vi "Read Decimal and Octal Label Tags.vi"(8 "error in":errorcluster, 11 "node in":refnum<k20>) -> (0 "error out":errorcluster, 1 "label (Dec)":u32, 2 "label (Display)":u32, 3 "node out":refnum<k20>)   [LabVIEW 2020, in "ARINC 429 Import.lvlib"]
uses:
  ARINC 429 Import.lvlib
  <vilib>/xml/NI_XML.lvlib
  <resource>/objmgr/DOMUserDefRef.rc
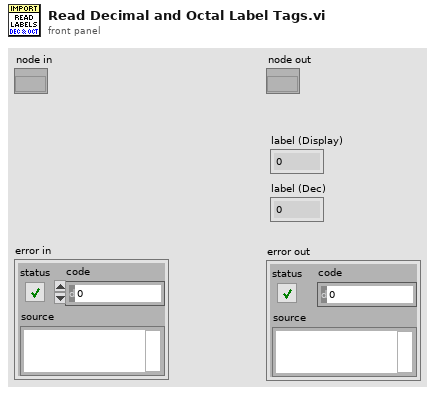
[diagram p1: front panel]
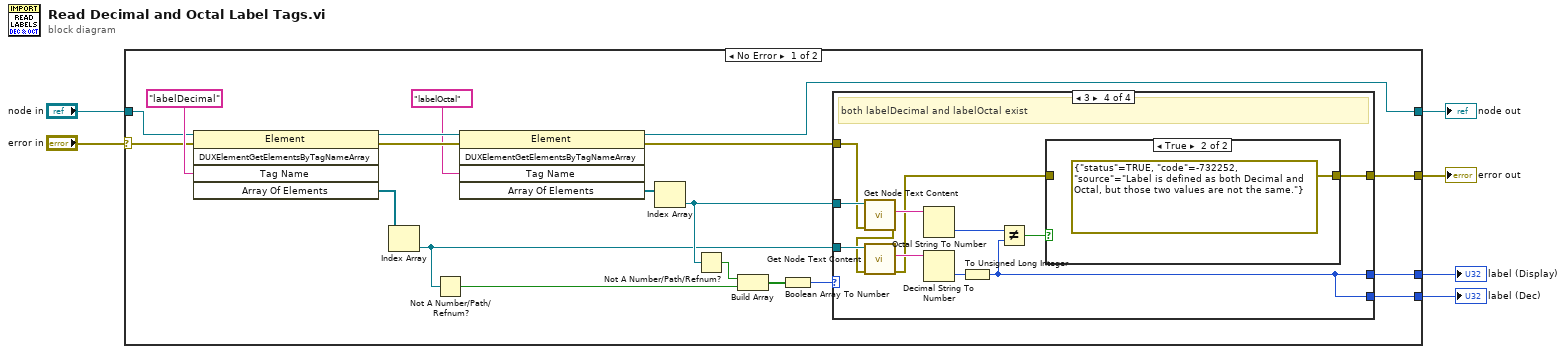
[diagram p0: block diagram]
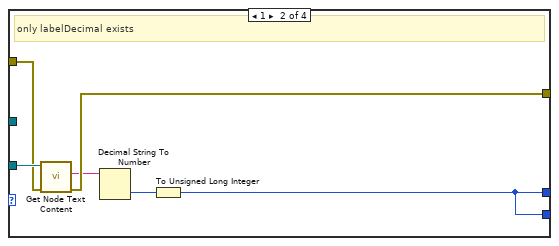
[diagram p3: hidden frame]
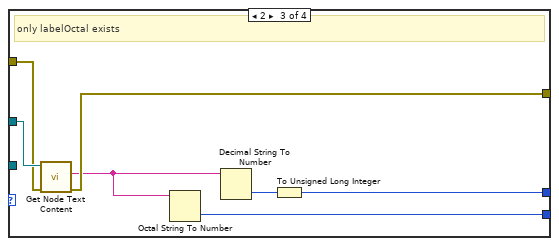
[diagram p4: hidden frame]
diagram:
  n1 = case shown="No Error" "error in" {
    selector: "error in" -> [w10 w55]
    tunnel: [w8 w55] -> w6
    tunnel: "node in" -> [w11 w54]
    tunnel: [w12 w54] -> w4
    tunnel: [w9 _] -> w2
    tunnel: [w7 _] -> w1
    frame No Error {
      n2 = invoke class="Element" method="DUXElementGetElementsByTagNameArray"(reference=w11, error in=w10, "Tag Name"="labelDecimal") -> (reference out=w17:refnum<k20>, error out=w18:errorcluster, "Array Of Elements"=w14:refnum<k20>[])  [unwired: 2 in, 2 out]
      n3 = Index Array(array=w14) -> (element=w23:refnum<k20>)  [unwired: 1 in]
      n4 = Not A Number/Path/Refnum?(number/path/refnum=w23) -> (NaN/Path/Refnum?=w20:bool)
      n5 = invoke class="Element" method="DUXElementGetElementsByTagNameArray"(reference=w17, error in=w18, "Tag Name"="labelOctal") -> (reference out=w12:refnum<k20>, error out=w25:errorcluster, "Array Of Elements"=w15:refnum<k20>[])  [unwired: 2 in, 2 out]
      n6 = Index Array(array=w15) -> (element=w24:refnum<k20>)  [unwired: 1 in]
      n7 = Not A Number/Path/Refnum?(number/path/refnum=w24) -> (NaN/Path/Refnum?=w19:bool)
      n8 = Build Array(w19, w20) -> (w21:bool[])
      n9 = Boolean Array To Number(Boolean array=w21) -> (number=w22:u32)
      n10 = case shown="3" w22 {
        tunnel: w23 -> [_ w32 _ w48]
        tunnel: w24 -> [_ _ w39 w49]
        tunnel: w25 -> [w26 w31 w38 w47]
        tunnel: [w26 w30 w37 w44] -> w8
        tunnel: [_ w28 w34 w40] -> w9
        tunnel: [_ w28 w35 w40] -> w7
        frame 0, Default {
          # "neither labelDecimal or labelOctal exist"
        }
        frame 1 {
          # "only labelDecimal exists"
          n11 = call <vilib>:"Get Node Text Content.vi"("error in (no error)"=w31, "node in"=w32) -> ("error out"=w30:errorcluster, "node text"=w27:string)  [unwired: 7 in, 1 out]
          n12 = Decimal String To Number(string=w27) -> (number=w29:i32)  [unwired: 2 in, 1 out]
          n13 = To Unsigned Long Integer(number=w29) -> (unsigned 32bit integer=w28:u32)
        }
        frame 2 {
          # "only labelOctal exists"
          n14 = call <vilib>:"Get Node Text Content.vi"("error in (no error)"=w38, "node in"=w39) -> ("error out"=w37:errorcluster, "node text"=w33:string)  [unwired: 7 in, 1 out]
          n15 = Octal String To Number(4:w33) -> (0:w35:u32)  [unwired: 2 in, 1 out]
          n16 = Decimal String To Number(string=w33) -> (number=w36:i32)  [unwired: 2 in, 1 out]
          n17 = To Unsigned Long Integer(number=w36) -> (unsigned 32bit integer=w34:u32)
        }
        frame 3 {
          # "both labelDecimal and labelOctal exist"
          n18 = call <vilib>:"Get Node Text Content.vi"("error in (no error)"=w47, "node in"=w49) -> ("error out"=w46:errorcluster, "node text"=w50:string)  [unwired: 7 in, 1 out]
          n19 = call <vilib>:"Get Node Text Content.vi"("error in (no error)"=w46, "node in"=w48) -> ("error out"=w43:errorcluster, "node text"=w51:string)  [unwired: 7 in, 1 out]
          n20 = Octal String To Number(4:w50) -> (0:w41:u32)  [unwired: 2 in, 1 out]
          n21 = Decimal String To Number(string=w51) -> (number=w45:i32)  [unwired: 2 in, 1 out]
          n22 = To Unsigned Long Integer(number=w45) -> (unsigned 32bit integer=w40:u32)
          n23 = Not Equal?(x=w41, y=w40) -> (x != y?=w42:bool)
          n24 = case shown="True" w42 {
            tunnel: [w52 errorcluster {"status"=TRUE, "code"=-732252, "source"="Label is defined as both Decimal and Octal, but those two values are not the same."} ("error constant")] -> w44
            tunnel: w43 -> [w52 _]
            frame False {
            }
            frame True {
            }
          }
        }
      }
    }
    frame Error {
    }
  }
  "error out" <- w6
  "node out" <- w4
  "label (Display)" <- w2
  "label (Dec)" <- w1
